vi "ActorDatabase-Initialize.vi"(8 "error in (no error)":errorcluster, 11 "Database-Actor In":refnum<class "Database-Actor.lvclass">) -> (0 "error out":errorcluster, 3 "Database-Actor out":refnum<class "Database-Actor.lvclass">)   [LabVIEW 2013, in "Database-Actor.lvclass"]
uses:
  Database-Actor.lvclass
  Database-Actor.lvclass/Database-Actor.ctl
  Reuse Library/Database API/Database-API.lvclass
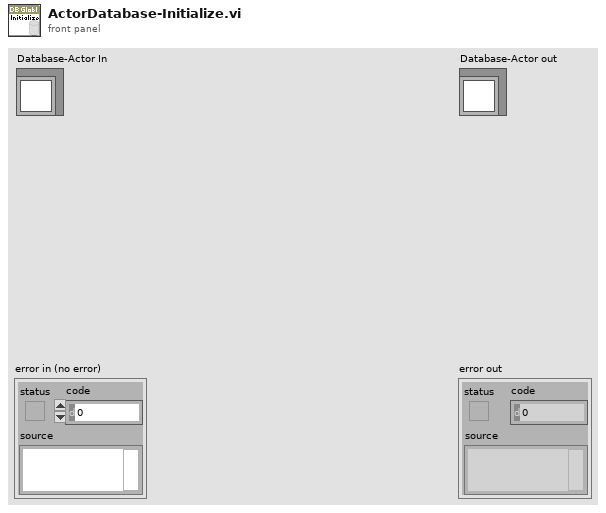
[diagram p1: front panel]
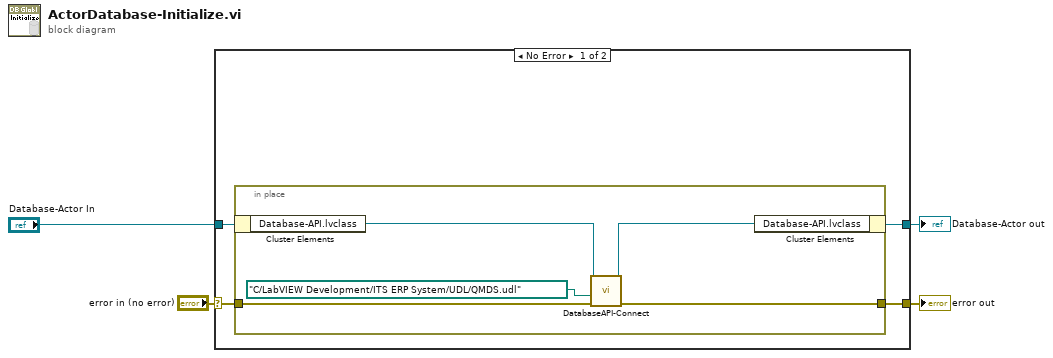
[diagram p0: block diagram]
diagram:
  n1 = case shown="No Error" "error in (no error)" {
    selector: "error in (no error)" -> [w7 w15]
    tunnel: [w6 w15] -> w3
    tunnel: [w8 w14] -> w2
    tunnel: "Database-Actor In" -> [w5 w14]
    frame No Error {
      n2 = in-place {
        in-place-border: w7 -> [w11]
        in-place-border: [w10] -> w6
        n3 = in-place-cluster #1(w5) -> ("Database-API.lvclass"=w13:refnum<class "Database-API.lvclass">)
        n4 = call "DatabaseAPI-Connect.vi"("error in (no error)"=w11, "Database (mdb)  File Path"=path "C:/LabVIEW Development/ITS ERP System/UDL/QMDS.udl", "Database-API in"=w13) -> ("error out"=w10:errorcluster, "Database-API out"=w12:refnum<class "Database-API.lvclass">)  [unwired: 7 in]
        n5 = in-place-cluster #1("Database-API.lvclass"=w12) -> (w8:refnum<class "Database-Actor.lvclass">)
      }
    }
    frame Error {
    }
  }
  "error out" <- w3
  "Database-Actor out" <- w2
